vi "Globals.vi"() -> ()   [LabVIEW 2012]
panel:
  out "Running":bool
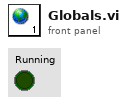
[diagram p1: front panel]
diagram:
